vi "HP 4275A Address constant.vi"() -> ()   [LabVIEW 2020]
uses:
  Control 1.ctl
panel:
  in  "HP 4275A Address":T1="3"
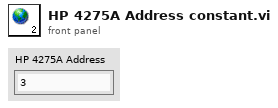
[diagram p1: front panel]
types:
  T1 = typedef "Control 1.ctl" = string
diagram:
